vi "Reset Row Hightlight.vi"(0 "Display State In":T1={"logTable"=refnum, "max items"=500, "displaydata"=[], "data"=[], "Auto Scroll"=TRUE, "current item"=500, "col headers"=[], "Add to Top"=TRUE, "Auto resize"=TRUE, "col size"=[], "filters"=[], "color cells"=[]}, 5 "Column":string, 7 "Value":string, 9 "Container State":T3, 11 "error in (no error)":errorcluster) -> (4 "Display State Out":T1={"logTable"=refnum, "max items"=500, "displaydata"=[], "data"=[], "Auto Scroll"=TRUE, "current item"=500, "col headers"=[], "Add to Top"=TRUE, "Auto resize"=TRUE, "col size"=[], "filters"=[], "color cells"=[]}, 15 "error out":errorcluster)   [LabVIEW 2017, in "UI-DisplayTable(dev).xctl"]
uses:
  UI-DisplayTable(dev).xctl
  <vilib>/_xctls/Container State.ctl
  State.ctl
  Support/DEF-Filter.ctl
  <vilib>/Utility/miscctls.llb/LVRowAndColumnTypeDef.ctl
  <vilib>/_xctls/XControlSupport.lvlib
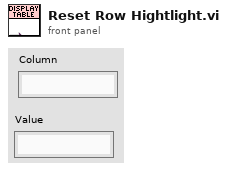
[diagram p1: front panel]
types:
  T1 = typedef "UI-DisplayTable(dev).xctl/State.ctl" = cluster{"logTable":refnum<vi>, "max items":i32, "displaydata":string[][], "data":string[][], "Auto Scroll":bool, "current item":i32, "col headers":string[], "Add to Top":bool, "Auto resize":bool, "col size":i32[], "filters":T2[], "color cells":cluster{"color cell":cluster{"Column":string, "Value":string, "Highlight Column":string}, "Color Box":u32}[]}
  T2 = typedef "UI-DisplayTable(dev).xctl/DEF-Filter.ctl" = cluster{"column":string, "value":string[]}
  T3 = typedef "XControlSupport.lvlib/Container State.ctl" = cluster{"Indicator?":bool, "Run Mode?":bool, " Refnum":refnum<vi>}
  T4 = typedef "LVRowAndColumnTypeDef.ctl" = cluster{"Row":i32, "Column":i32}
  T5 = cluster{"color cell":cluster{"Column":string, "Value":string, "Highlight Column":string}, "Color Box":u32}[]
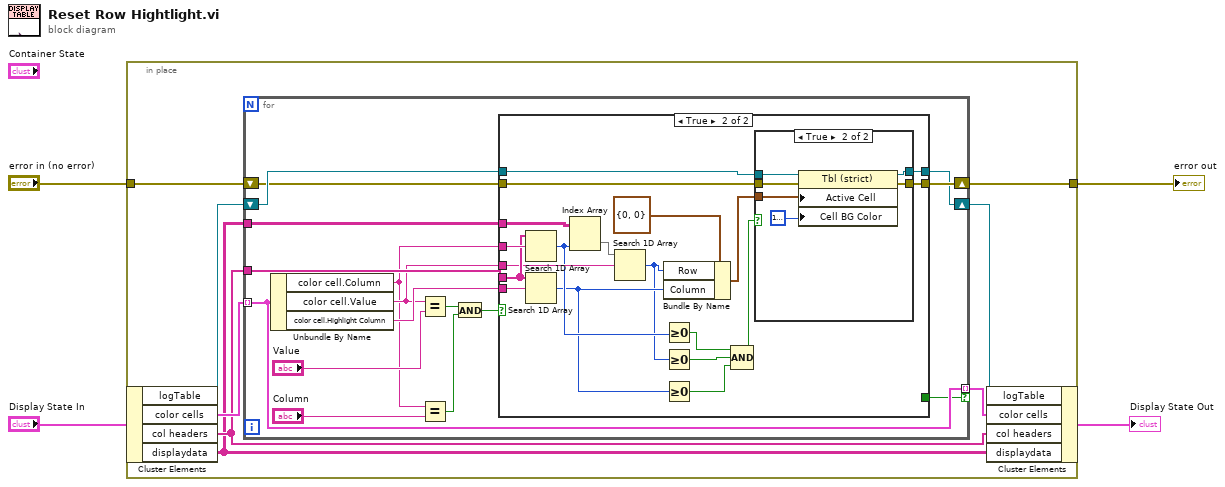
[diagram p0: block diagram]
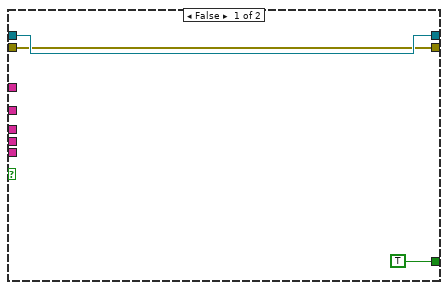
[diagram p2: hidden frame]
diagram:
  n1 = in-place {
    in-place-border: "error in (no error)" -> [w12]
    in-place-border: [w11] -> w3
    n2 = in-place-cluster #1("Display State In") -> ("logTable"=w9:refnum<vi>, "color cells"=w10:T5, "col headers"=w7:string[], "displaydata"=w6:string[][])
    n3 = for {
      tunnel: w10 -> [w21] mode=indexing
      shift-right: [w26] -> w11
      shift-left: w12 -> [w27]
      tunnel: w7 -> [w23]
      tunnel: w6 -> [w25]
      shift-right: [w22] -> w8
      shift-left: w9 -> [w28]
      tunnel: [w21] -> w5 mode=indexing if=w20
      n4 = Unbundle By Name(w21) -> ("color cell.Column"=w13:string, "color cell.Value"=w14:string, "color cell.Highlight Column"=w24:string)
      n5 = Equal?(x=w14, y="Value") -> (x = y?=w16:bool)
      n6 = Equal?(x=w13, y="Column") -> (x = y?=w17:bool)
      n7 = And(x=w16, y=w17) -> (x .and. y?=w15:bool)
      n8 = case shown="True" w15 {
        tunnel: w28 -> [w31 w50]
        tunnel: w27 -> [w30 w49]
        tunnel: [w30 w48] -> w26
        tunnel: w13 -> [_ w47]
        tunnel: w25 -> [_ w46]
        tunnel: w24 -> [_ w45]
        tunnel: w23 -> [_ w44]
        tunnel: w14 -> [_ w43]
        tunnel: [w31 w39] -> w22
        tunnel: [TRUE _] -> w20
        frame False {
        }
        frame True {
          n9 = Search 1D Array(1D array=w44, element=w47) -> (index of element=w38:i32)  [unwired: 1 in]
          n10 = Search 1D Array(1D array=w44, element=w45) -> (index of element=w37:i32)  [unwired: 1 in]
          n11 = Index Array(array=w46, index (col)=w38) -> (element=w42:string[])  [unwired: 1 in]
          n12 = Search 1D Array(1D array=w42, element=w43) -> (index of element=w36:i32)  [unwired: 1 in]
          n13 = Bundle By Name(cluster=T4 {"Row"=0, "Column"=0} ("Active Cell:Active Cell"), "Row"=w36, "Column"=w37) -> (w40:T4)
          n14 = Greater Or Equal To 0?(x=w38) -> (x >= 0?=w35:bool)
          n15 = Greater Or Equal To 0?(x=w36) -> (x >= 0?=w34:bool)
          n16 = Greater Or Equal To 0?(x=w37) -> (x >= 0?=w33:bool)
          n17 = Compound Arithmetic op=AND(w35, w34, w33) -> (w32:bool)
          n18 = case shown="True" w32 {
            tunnel: w50 -> [w52 w58]
            tunnel: w49 -> [w51 w57]
            tunnel: [w51 w56] -> w48
            tunnel: w40 -> [_ w55]
            tunnel: [w52 w54] -> w39
            frame False {
            }
            frame True {
              n19 = property class="Tbl (strict)"(reference=w58, error in=w57, "Active Cell"=w55, "Cell BG Color"=u32 16777216 ("Active Cell:Cell Background Color")) -> (reference out=w54:refnum<vi>, error out=w56:errorcluster)
            }
          }
        }
      }
    }
    n20 = in-place-cluster #1("logTable"=w8, "color cells"=w5, "col headers"=w7, "displaydata"=w6) -> (→"Display State Out":T1)
  }
  "error out" <- w3
